vi "GetEventForceSetpointWarningField.vi"(10 "Event Data":string, 11 "Cluster in":refnum<vi>) -> (3 "Array":string[](array[string]))   [LabVIEW 2016]
uses:
  SALLV_m1m3/DataTypes/logevent_ForceSetpointWarning.ctl
  SALLV_m1m3/SALLV_m1m3.lvlib
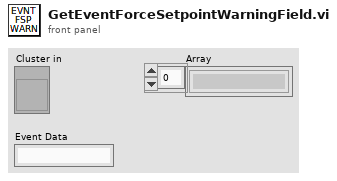
[diagram p1: front panel]
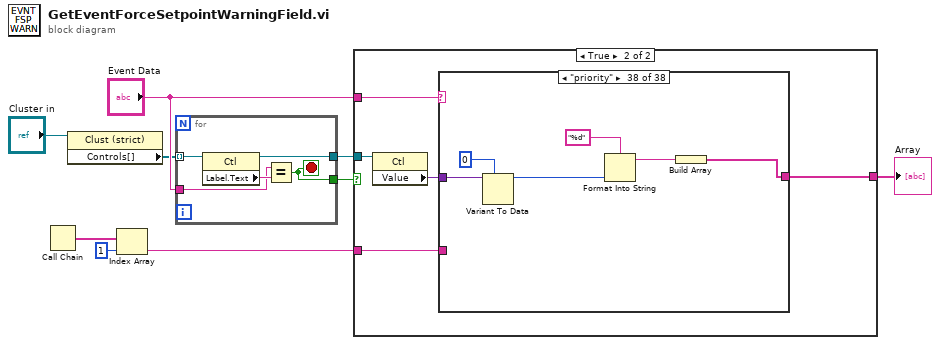
[diagram p0: block diagram]
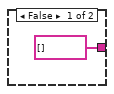
[diagram p2: hidden frame]
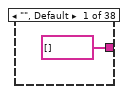
[diagram p3: hidden frame]
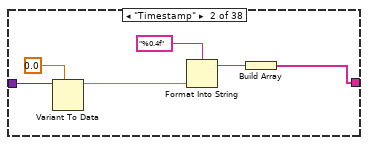
[diagram p4: hidden frame]
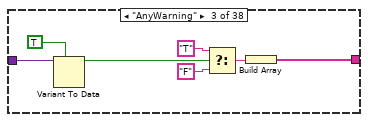
[diagram p5: hidden frame]
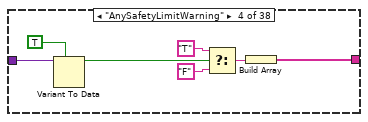
[diagram p6: hidden frame]
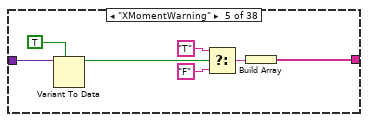
[diagram p7: hidden frame]
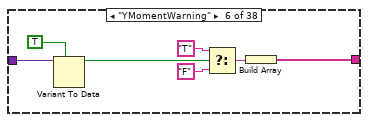
[diagram p8: hidden frame]
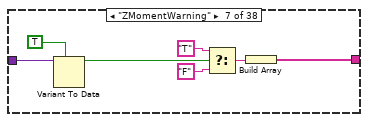
[diagram p9: hidden frame]
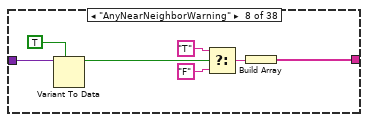
[diagram p10: hidden frame]
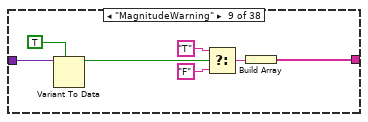
[diagram p11: hidden frame]
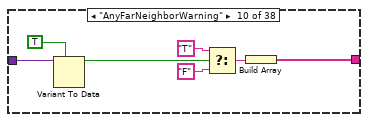
[diagram p12: hidden frame]
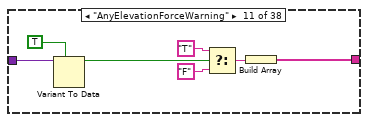
[diagram p13: hidden frame]
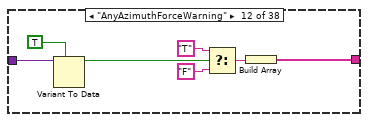
[diagram p14: hidden frame]
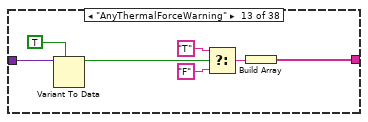
[diagram p15: hidden frame]
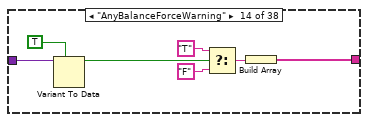
[diagram p16: hidden frame]
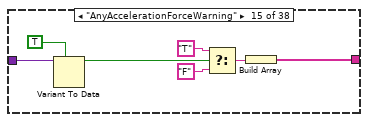
[diagram p17: hidden frame]
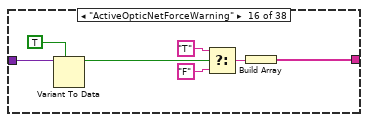
[diagram p18: hidden frame]
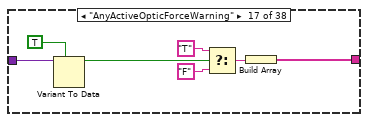
[diagram p19: hidden frame]
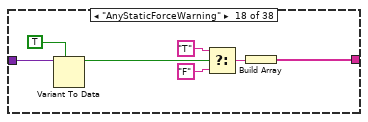
[diagram p20: hidden frame]
diagram:
  n1 = Call Chain() -> (call chain=w2:string[])
  n2 = property on="Property Node" class="Clust (strict)"(reference="Cluster in") -> ("Controls[]"=w6:refnum<vi>[])  [unwired: 1 in, 2 out]
  n3 = Index Array(array=w2, index=1) -> (element=w1:string)
  n4 = for {
    tunnel: w6 -> [w14] mode=indexing
    tunnel: [w13] -> w8
    tunnel: "Event Data" -> [w11]
    tunnel: [w10] -> w9
    stop <- w10 stop-if-true
    n5 = property on="Property Node" class="Ctl"(reference=w14) -> (reference out=w13:refnum<vi>, "Label.Text"=w12:string)  [unwired: 1 in, 1 out]
    n6 = Equal?(x=w11, y=w12) -> (x = y?=w10:bool)
  }
  n7 = case shown="True" w9 {
    tunnel: "Event Data" -> [_ w20]
    tunnel: w8 -> [_ w19]
    tunnel: [string[] [] w17] -> w5
    tunnel: w1 -> [_ w16]
    frame False {
    }
    frame True {
      n8 = property on="Property Node" class="Ctl"(reference=w19) -> ("Value"=w18:variant)  [unwired: 1 in, 2 out]
      n9 = case shown="\"priority\"" w20 {
        tunnel: [string[] [] w25 w28 w35 w42 w49 w56 w63 w70 w77 w84 w91 w98 w105 w112 w119 w126 w133 w140 w147 w154 w161 w168 w176 w192 w208 w224 w240 w256 w272 w288 w304 w320 w336 w352 w368 w384 w402] -> w17
        tunnel: w18 -> [_ w23 w34 w41 w48 w55 w62 w69 w76 w83 w90 w97 w104 w111 w118 w125 w132 w139 w146 w153 w160 w167 w174 w179 w195 w211 w227 w243 w259 w275 w291 w307 w323 w339 w355 w371 w387 w400]
        tunnel: w16 -> [_ _ _ _ _ _ _ _ _ _ _ _ _ _ _ _ _ _ _ _ _ _ _ w175 w191 w207 w223 w239 w255 w271 w287 w303 w319 w335 w351 w367 w383 _]
        frame "", Default {
        }
        frame "Timestamp" {
          n10 = Variant To Data(type=0.0, Variant=w23) -> (data=w24:dbl)  [unwired: 1 in, 1 out]
          n11 = Format Into String(format string="%0.4f", w24) -> (resulting string=w26:string)  [unwired: 2 in, 1 out]
          n12 = Build Array(w26) -> (w25:string[])
        }
        frame "AnyWarning" {
          n13 = Variant To Data(type=TRUE, Variant=w34) -> (data=w32:bool)  [unwired: 1 in, 1 out]
          n14 = Select(t="T", s=w32, f="F") -> (s? t:f=w29:string)
          n15 = Build Array(w29) -> (w28:string[])
        }
        frame "AnySafetyLimitWarning" {
          n16 = Variant To Data(type=TRUE, Variant=w41) -> (data=w39:bool)  [unwired: 1 in, 1 out]
          n17 = Select(t="T", s=w39, f="F") -> (s? t:f=w36:string)
          n18 = Build Array(w36) -> (w35:string[])
        }
        frame "XMomentWarning" {
          n19 = Variant To Data(type=TRUE, Variant=w48) -> (data=w46:bool)  [unwired: 1 in, 1 out]
          n20 = Select(t="T", s=w46, f="F") -> (s? t:f=w43:string)
          n21 = Build Array(w43) -> (w42:string[])
        }
        frame "YMomentWarning" {
          n22 = Variant To Data(type=TRUE, Variant=w55) -> (data=w53:bool)  [unwired: 1 in, 1 out]
          n23 = Select(t="T", s=w53, f="F") -> (s? t:f=w50:string)
          n24 = Build Array(w50) -> (w49:string[])
        }
        frame "ZMomentWarning" {
          n25 = Variant To Data(type=TRUE, Variant=w62) -> (data=w60:bool)  [unwired: 1 in, 1 out]
          n26 = Select(t="T", s=w60, f="F") -> (s? t:f=w57:string)
          n27 = Build Array(w57) -> (w56:string[])
        }
        frame "AnyNearNeighborWarning" {
          n28 = Variant To Data(type=TRUE, Variant=w69) -> (data=w67:bool)  [unwired: 1 in, 1 out]
          n29 = Select(t="T", s=w67, f="F") -> (s? t:f=w64:string)
          n30 = Build Array(w64) -> (w63:string[])
        }
        frame "MagnitudeWarning" {
          n31 = Variant To Data(type=TRUE, Variant=w76) -> (data=w74:bool)  [unwired: 1 in, 1 out]
          n32 = Select(t="T", s=w74, f="F") -> (s? t:f=w71:string)
          n33 = Build Array(w71) -> (w70:string[])
        }
        frame "AnyFarNeighborWarning" {
          n34 = Variant To Data(type=TRUE, Variant=w83) -> (data=w81:bool)  [unwired: 1 in, 1 out]
          n35 = Select(t="T", s=w81, f="F") -> (s? t:f=w78:string)
          n36 = Build Array(w78) -> (w77:string[])
        }
        frame "AnyElevationForceWarning" {
          n37 = Variant To Data(type=TRUE, Variant=w90) -> (data=w88:bool)  [unwired: 1 in, 1 out]
          n38 = Select(t="T", s=w88, f="F") -> (s? t:f=w85:string)
          n39 = Build Array(w85) -> (w84:string[])
        }
        frame "AnyAzimuthForceWarning" {
          n40 = Variant To Data(type=TRUE, Variant=w97) -> (data=w95:bool)  [unwired: 1 in, 1 out]
          n41 = Select(t="T", s=w95, f="F") -> (s? t:f=w92:string)
          n42 = Build Array(w92) -> (w91:string[])
        }
        frame "AnyThermalForceWarning" {
          n43 = Variant To Data(type=TRUE, Variant=w104) -> (data=w102:bool)  [unwired: 1 in, 1 out]
          n44 = Select(t="T", s=w102, f="F") -> (s? t:f=w99:string)
          n45 = Build Array(w99) -> (w98:string[])
        }
        frame "AnyBalanceForceWarning" {
          n46 = Variant To Data(type=TRUE, Variant=w111) -> (data=w109:bool)  [unwired: 1 in, 1 out]
          n47 = Select(t="T", s=w109, f="F") -> (s? t:f=w106:string)
          n48 = Build Array(w106) -> (w105:string[])
        }
        frame "AnyAccelerationForceWarning" {
          n49 = Variant To Data(type=TRUE, Variant=w118) -> (data=w116:bool)  [unwired: 1 in, 1 out]
          n50 = Select(t="T", s=w116, f="F") -> (s? t:f=w113:string)
          n51 = Build Array(w113) -> (w112:string[])
        }
        frame "ActiveOpticNetForceWarning" {
          n52 = Variant To Data(type=TRUE, Variant=w125) -> (data=w123:bool)  [unwired: 1 in, 1 out]
          n53 = Select(t="T", s=w123, f="F") -> (s? t:f=w120:string)
          n54 = Build Array(w120) -> (w119:string[])
        }
        frame "AnyActiveOpticForceWarning" {
          n55 = Variant To Data(type=TRUE, Variant=w132) -> (data=w130:bool)  [unwired: 1 in, 1 out]
          n56 = Select(t="T", s=w130, f="F") -> (s? t:f=w127:string)
          n57 = Build Array(w127) -> (w126:string[])
        }
        frame "AnyStaticForceWarning" {
          n58 = Variant To Data(type=TRUE, Variant=w139) -> (data=w137:bool)  [unwired: 1 in, 1 out]
          n59 = Select(t="T", s=w137, f="F") -> (s? t:f=w134:string)
          n60 = Build Array(w134) -> (w133:string[])
        }
        frame "AberrationNetForceWarning" {
          n61 = Variant To Data(type=TRUE, Variant=w146) -> (data=w144:bool)  [unwired: 1 in, 1 out]
          n62 = Select(t="T", s=w144, f="F") -> (s? t:f=w141:string)
          n63 = Build Array(w141) -> (w140:string[])
        }
        frame "AnyAberrationForceWarning" {
          n64 = Variant To Data(type=TRUE, Variant=w153) -> (data=w151:bool)  [unwired: 1 in, 1 out]
          n65 = Select(t="T", s=w151, f="F") -> (s? t:f=w148:string)
          n66 = Build Array(w148) -> (w147:string[])
        }
        frame "AnyOffsetForceWarning" {
          n67 = Variant To Data(type=TRUE, Variant=w160) -> (data=w158:bool)  [unwired: 1 in, 1 out]
          n68 = Select(t="T", s=w158, f="F") -> (s? t:f=w155:string)
          n69 = Build Array(w155) -> (w154:string[])
        }
        frame "AnyVelocityForceWarning" {
          n70 = Variant To Data(type=TRUE, Variant=w167) -> (data=w165:bool)  [unwired: 1 in, 1 out]
          n71 = Select(t="T", s=w165, f="F") -> (s? t:f=w162:string)
          n72 = Build Array(w162) -> (w161:string[])
        }
        frame "AnyForceWarning" {
          n73 = Variant To Data(type=TRUE, Variant=w174) -> (data=w172:bool)  [unwired: 1 in, 1 out]
          n74 = Select(t="T", s=w172, f="F") -> (s? t:f=w169:string)
          n75 = Build Array(w169) -> (w168:string[])
        }
        frame "SafetyLimitWarning[156]" {
          n76 = Variant To Data(type=bool[] [], Variant=w179) -> (data=w177:bool[])  [unwired: 1 in, 1 out]
          n77 = for {
            tunnel: w177 -> [w181] mode=indexing
            tunnel: [w180] -> w176 mode=indexing
            tunnel: w175 -> [w182]
            n78 = case shown="\"M1M3SupportEUI_Views.lvlib:FA Graphic View.vi\"" w182 {
              tunnel: w181 -> [w186 w190]
              tunnel: [w185 w187] -> w180
              frame "M1M3SupportEUI_Views.lvlib:FA Graphic View.vi" {
                n79 = Select(t="1", s=w186, f="0") -> (s? t:f=w185:string)
              }
              frame "", Default {
                n80 = Select(t="T", s=w190, f="F") -> (s? t:f=w187:string)
              }
            }
          }
        }
        frame "NearNeighborWarning[156]" {
          n81 = Variant To Data(type=bool[] [], Variant=w195) -> (data=w193:bool[])  [unwired: 1 in, 1 out]
          n82 = for {
            tunnel: w193 -> [w198] mode=indexing
            tunnel: [w197] -> w192 mode=indexing
            tunnel: w191 -> [w196]
            n83 = case shown="\"M1M3SupportEUI_Views.lvlib:FA Graphic View.vi\"" w196 {
              tunnel: w198 -> [w202 w206]
              tunnel: [w201 w203] -> w197
              frame "M1M3SupportEUI_Views.lvlib:FA Graphic View.vi" {
                n84 = Select(t="1", s=w202, f="0") -> (s? t:f=w201:string)
              }
              frame "", Default {
                n85 = Select(t="T", s=w206, f="F") -> (s? t:f=w203:string)
              }
            }
          }
        }
        frame "FarNeighborWarning[156]" {
          n86 = Variant To Data(type=bool[] [], Variant=w211) -> (data=w209:bool[])  [unwired: 1 in, 1 out]
          n87 = for {
            tunnel: w209 -> [w214] mode=indexing
            tunnel: [w213] -> w208 mode=indexing
            tunnel: w207 -> [w212]
            n88 = case shown="\"M1M3SupportEUI_Views.lvlib:FA Graphic View.vi\"" w212 {
              tunnel: w214 -> [w218 w222]
              tunnel: [w217 w219] -> w213
              frame "M1M3SupportEUI_Views.lvlib:FA Graphic View.vi" {
                n89 = Select(t="1", s=w218, f="0") -> (s? t:f=w217:string)
              }
              frame "", Default {
                n90 = Select(t="T", s=w222, f="F") -> (s? t:f=w219:string)
              }
            }
          }
        }
        frame "ElevationForceWarning[156]" {
          n91 = Variant To Data(type=bool[] [], Variant=w227) -> (data=w225:bool[])  [unwired: 1 in, 1 out]
          n92 = for {
            tunnel: w225 -> [w230] mode=indexing
            tunnel: [w229] -> w224 mode=indexing
            tunnel: w223 -> [w228]
            n93 = case shown="\"M1M3SupportEUI_Views.lvlib:FA Graphic View.vi\"" w228 {
              tunnel: w230 -> [w234 w238]
              tunnel: [w233 w235] -> w229
              frame "M1M3SupportEUI_Views.lvlib:FA Graphic View.vi" {
                n94 = Select(t="1", s=w234, f="0") -> (s? t:f=w233:string)
              }
              frame "", Default {
                n95 = Select(t="T", s=w238, f="F") -> (s? t:f=w235:string)
              }
            }
          }
        }
        frame "AzimuthForceWarning[156]" {
          n96 = Variant To Data(type=bool[] [], Variant=w243) -> (data=w241:bool[])  [unwired: 1 in, 1 out]
          n97 = for {
            tunnel: w241 -> [w246] mode=indexing
            tunnel: [w245] -> w240 mode=indexing
            tunnel: w239 -> [w244]
            n98 = case shown="\"M1M3SupportEUI_Views.lvlib:FA Graphic View.vi\"" w244 {
              tunnel: w246 -> [w250 w254]
              tunnel: [w249 w251] -> w245
              frame "M1M3SupportEUI_Views.lvlib:FA Graphic View.vi" {
                n99 = Select(t="1", s=w250, f="0") -> (s? t:f=w249:string)
              }
              frame "", Default {
                n100 = Select(t="T", s=w254, f="F") -> (s? t:f=w251:string)
              }
            }
          }
        }
        frame "ThermalForceWarning[156]" {
          n101 = Variant To Data(type=bool[] [], Variant=w259) -> (data=w257:bool[])  [unwired: 1 in, 1 out]
          n102 = for {
            tunnel: w257 -> [w261] mode=indexing
            tunnel: [w262] -> w256 mode=indexing
            tunnel: w255 -> [w260]
            n103 = case shown="\"M1M3SupportEUI_Views.lvlib:FA Graphic View.vi\"" w260 {
              tunnel: w261 -> [w266 w270]
              tunnel: [w265 w267] -> w262
              frame "M1M3SupportEUI_Views.lvlib:FA Graphic View.vi" {
                n104 = Select(t="1", s=w266, f="0") -> (s? t:f=w265:string)
              }
              frame "", Default {
                n105 = Select(t="T", s=w270, f="F") -> (s? t:f=w267:string)
              }
            }
          }
        }
        frame "BalanceForceWarning[156]" {
          n106 = Variant To Data(type=bool[] [], Variant=w275) -> (data=w273:bool[])  [unwired: 1 in, 1 out]
          n107 = for {
            tunnel: w273 -> [w278] mode=indexing
            tunnel: [w277] -> w272 mode=indexing
            tunnel: w271 -> [w276]
            n108 = case shown="\"M1M3SupportEUI_Views.lvlib:FA Graphic View.vi\"" w276 {
              tunnel: w278 -> [w282 w286]
              tunnel: [w281 w283] -> w277
              frame "M1M3SupportEUI_Views.lvlib:FA Graphic View.vi" {
                n109 = Select(t="1", s=w282, f="0") -> (s? t:f=w281:string)
              }
              frame "", Default {
                n110 = Select(t="T", s=w286, f="F") -> (s? t:f=w283:string)
              }
            }
          }
        }
        frame "AccelerationForceWarning[156]" {
          n111 = Variant To Data(type=bool[] [], Variant=w291) -> (data=w289:bool[])  [unwired: 1 in, 1 out]
          n112 = for {
            tunnel: w289 -> [w294] mode=indexing
            tunnel: [w293] -> w288 mode=indexing
            tunnel: w287 -> [w292]
            n113 = case shown="\"M1M3SupportEUI_Views.lvlib:FA Graphic View.vi\"" w292 {
              tunnel: w294 -> [w298 w302]
              tunnel: [w297 w299] -> w293
              frame "M1M3SupportEUI_Views.lvlib:FA Graphic View.vi" {
                n114 = Select(t="1", s=w298, f="0") -> (s? t:f=w297:string)
              }
              frame "", Default {
                n115 = Select(t="T", s=w302, f="F") -> (s? t:f=w299:string)
              }
            }
          }
        }
        frame "ActiveOpticForceWarning[156]" {
          n116 = Variant To Data(type=bool[] [], Variant=w307) -> (data=w305:bool[])  [unwired: 1 in, 1 out]
          n117 = for {
            tunnel: w305 -> [w310] mode=indexing
            tunnel: [w309] -> w304 mode=indexing
            tunnel: w303 -> [w308]
            n118 = case shown="\"M1M3SupportEUI_Views.lvlib:FA Graphic View.vi\"" w308 {
              tunnel: w310 -> [w314 w318]
              tunnel: [w313 w315] -> w309
              frame "M1M3SupportEUI_Views.lvlib:FA Graphic View.vi" {
                n119 = Select(t="1", s=w314, f="0") -> (s? t:f=w313:string)
              }
              frame "", Default {
                n120 = Select(t="T", s=w318, f="F") -> (s? t:f=w315:string)
              }
            }
          }
        }
        frame "StaticForceWarning[156]" {
          n121 = Variant To Data(type=bool[] [], Variant=w323) -> (data=w321:bool[])  [unwired: 1 in, 1 out]
          n122 = for {
            tunnel: w321 -> [w326] mode=indexing
            tunnel: [w325] -> w320 mode=indexing
            tunnel: w319 -> [w324]
            n123 = case shown="\"M1M3SupportEUI_Views.lvlib:FA Graphic View.vi\"" w324 {
              tunnel: w326 -> [w330 w334]
              tunnel: [w329 w331] -> w325
              frame "M1M3SupportEUI_Views.lvlib:FA Graphic View.vi" {
                n124 = Select(t="1", s=w330, f="0") -> (s? t:f=w329:string)
              }
              frame "", Default {
                n125 = Select(t="T", s=w334, f="F") -> (s? t:f=w331:string)
              }
            }
          }
        }
        frame "AberrationForceWarning[156]" {
          n126 = Variant To Data(type=bool[] [], Variant=w339) -> (data=w337:bool[])  [unwired: 1 in, 1 out]
          n127 = for {
            tunnel: w337 -> [w342] mode=indexing
            tunnel: [w341] -> w336 mode=indexing
            tunnel: w335 -> [w340]
            n128 = case shown="\"M1M3SupportEUI_Views.lvlib:FA Graphic View.vi\"" w340 {
              tunnel: w342 -> [w346 w350]
              tunnel: [w345 w347] -> w341
              frame "M1M3SupportEUI_Views.lvlib:FA Graphic View.vi" {
                n129 = Select(t="1", s=w346, f="0") -> (s? t:f=w345:string)
              }
              frame "", Default {
                n130 = Select(t="T", s=w350, f="F") -> (s? t:f=w347:string)
              }
            }
          }
        }
        frame "OffsetForceWarning[156]" {
          n131 = Variant To Data(type=bool[] [], Variant=w355) -> (data=w353:bool[])  [unwired: 1 in, 1 out]
          n132 = for {
            tunnel: w353 -> [w358] mode=indexing
            tunnel: [w357] -> w352 mode=indexing
            tunnel: w351 -> [w356]
            n133 = case shown="\"M1M3SupportEUI_Views.lvlib:FA Graphic View.vi\"" w356 {
              tunnel: w358 -> [w362 w366]
              tunnel: [w361 w363] -> w357
              frame "M1M3SupportEUI_Views.lvlib:FA Graphic View.vi" {
                n134 = Select(t="1", s=w362, f="0") -> (s? t:f=w361:string)
              }
              frame "", Default {
                n135 = Select(t="T", s=w366, f="F") -> (s? t:f=w363:string)
              }
            }
          }
        }
        frame "VelocityForceWarning[156]" {
          n136 = Variant To Data(type=bool[] [], Variant=w371) -> (data=w369:bool[])  [unwired: 1 in, 1 out]
          n137 = for {
            tunnel: w369 -> [w374] mode=indexing
            tunnel: [w373] -> w368 mode=indexing
            tunnel: w367 -> [w372]
            n138 = case shown="\"M1M3SupportEUI_Views.lvlib:FA Graphic View.vi\"" w372 {
              tunnel: w374 -> [w378 w382]
              tunnel: [w377 w379] -> w373
              frame "M1M3SupportEUI_Views.lvlib:FA Graphic View.vi" {
                n139 = Select(t="1", s=w378, f="0") -> (s? t:f=w377:string)
              }
              frame "", Default {
                n140 = Select(t="T", s=w382, f="F") -> (s? t:f=w379:string)
              }
            }
          }
        }
        frame "ForceWarning[156]" {
          n141 = Variant To Data(type=bool[] [], Variant=w387) -> (data=w385:bool[])  [unwired: 1 in, 1 out]
          n142 = for {
            tunnel: w385 -> [w390] mode=indexing
            tunnel: [w389] -> w384 mode=indexing
            tunnel: w383 -> [w388]
            n143 = case shown="\"M1M3SupportEUI_Views.lvlib:FA Graphic View.vi\"" w388 {
              tunnel: w390 -> [w394 w398]
              tunnel: [w393 w395] -> w389
              frame "M1M3SupportEUI_Views.lvlib:FA Graphic View.vi" {
                n144 = Select(t="1", s=w394, f="0") -> (s? t:f=w393:string)
              }
              frame "", Default {
                n145 = Select(t="T", s=w398, f="F") -> (s? t:f=w395:string)
              }
            }
          }
        }
        frame "priority" {
          n146 = Variant To Data(type=0, Variant=w400) -> (data=w401:i32)  [unwired: 1 in, 1 out]
          n147 = Format Into String(format string="%d", w401) -> (resulting string=w403:string)  [unwired: 2 in, 1 out]
          n148 = Build Array(w403) -> (w402:string[])
        }
      }
    }
  }
  "Array" <- w5
